vi "iV programa 2_4.vi"() -> ()   [LabVIEW 2020]
panel:
  in  "Operacion":T1(ring)
  in  "stop":bool
  out "?":dbl
  out "String":string="El resultado de A / B es: "
  in  "B":dbl
  in  "A":dbl
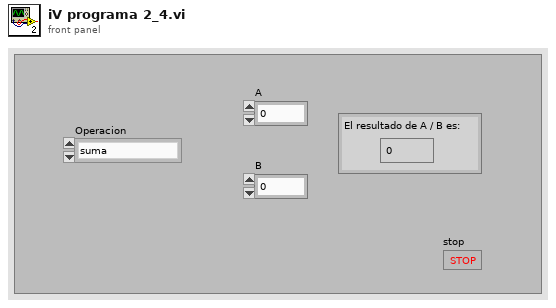
[diagram p1: front panel]
types:
  T1 = enum16{"suma", "resta", "multiplicacion", "divicion"}
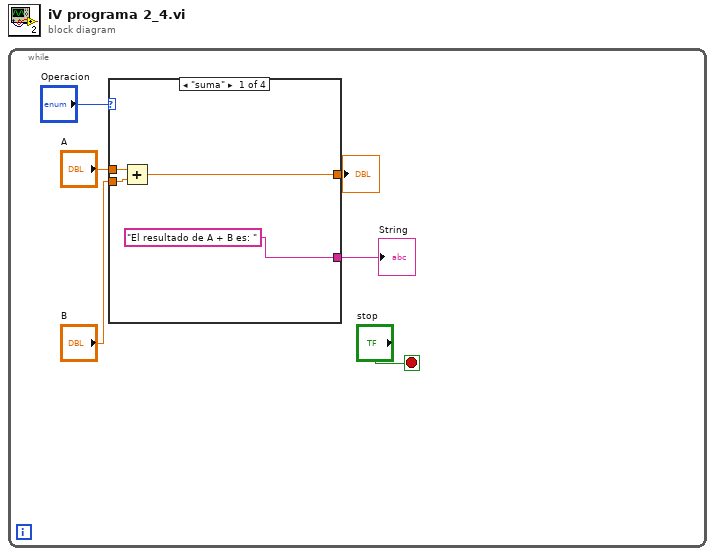
[diagram p0: block diagram]
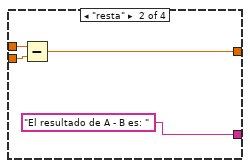
[diagram p2: hidden frame]
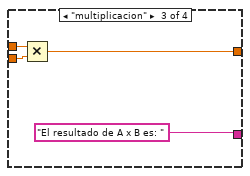
[diagram p3: hidden frame]
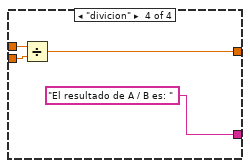
[diagram p4: hidden frame]
diagram:
  n1 = while {
    stop <- "stop" stop-if-true
    n2 = case shown="\"suma\"" "Operacion" {
      tunnel: "A" -> [w10 w14 w18 w22]
      tunnel: "B" -> [w9 w13 w17 w21]
      tunnel: [w8 w12 w16 w20] -> w3
      tunnel: ["El resultado de A + B es: " "El resultado de A - B es: " "El resultado de A x B es: " "El resultado de A / B es: "] -> w1
      frame "suma" {
        n3 = Add(x=w10, y=w9) -> (x+y=w8:dbl)
      }
      frame "resta" {
        n4 = Subtract(x=w14, y=w13) -> (x-y=w12:dbl)
      }
      frame "multiplicacion" {
        n5 = Multiply(x=w18, y=w17) -> (x*y=w16:dbl)
      }
      frame "divicion" {
        n6 = Divide(x=w22, y=w21) -> (x/y=w20:dbl)
      }
    }
    "?" <- w3
    "String" <- w1
  }
